vi "Tree Is Open For Edit.vi"(8 "error in (no error)":errorcluster, 11 "Tree DVR in":refnum<data-value>) -> (0 "error out":errorcluster, 2 "Is open for edit?":bool, 3 "Tree DVR out":refnum<data-value>)   [LabVIEW 2010, in "MDSplus.lvlib"]
uses:
  <vilib>/MDSplus/Library/MDSplus.lvlib
  <vilib>/MDSplus/Classes/Tree_Class/Tree.lvclass
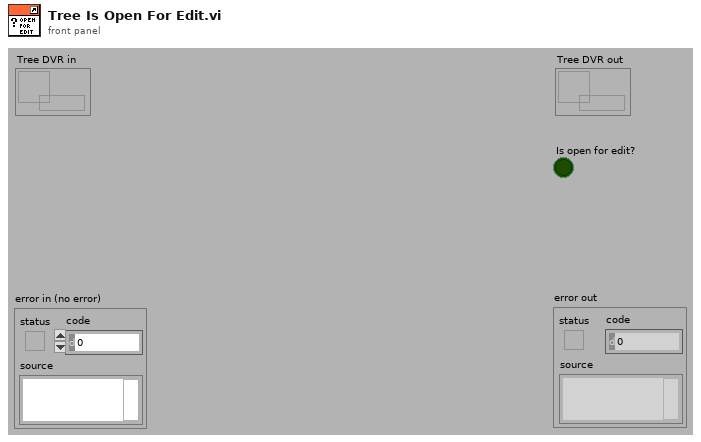
[diagram p1: front panel]
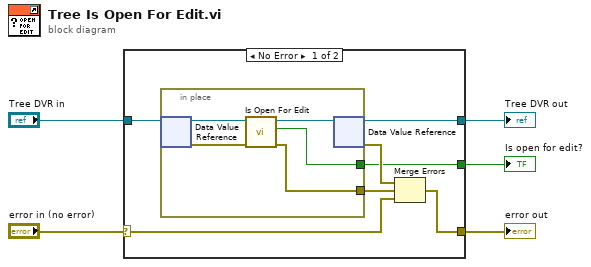
[diagram p0: block diagram]
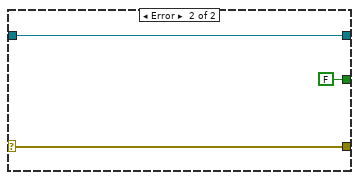
[diagram p2: hidden frame]
diagram:
  n1 = case shown="No Error" "error in (no error)" {
    selector: "error in (no error)" -> [w11 w20]
    tunnel: "Tree DVR in" -> [w12 w19]
    tunnel: [w9 w20] -> w5
    tunnel: [w8 w19] -> w2
    tunnel: [w6 FALSE ("Is modified?")] -> w1
    frame No Error {
      n2 = in-place {
        in-place-border: [w14] -> w7
        in-place-border: [w13] -> w6
        n3 = in-place-dvr #1(w12) -> (w17:refnum<class "Tree.lvclass">, w15:errorcluster)
        n4 = call-dynamic "Is Open For Edit.vi"("error in (no error)"=w15, "Tree in"=w17) -> ("error out"=w14:errorcluster, "Is open for edit?"=w13:bool, "Tree out"=w16:refnum<class "Tree.lvclass">)  [unwired: 7 in]
        n5 = in-place-dvr #1(w16) -> (w8:refnum<data-value>, w10:errorcluster)
      }
      n6 = Merge Errors(w10, w7, w11) -> (w9:errorcluster)
    }
    frame Error {
    }
  }
  "error out" <- w5
  "Tree DVR out" <- w2
  "Is open for edit?" <- w1
